vi "sedSpectrometer_flushSamplesEvent_ErrorCode.vi"(8 "error in (no error)":errorcluster) -> (0 "error out":errorcluster, 3 "function return":i32)   [LabVIEW 2016, in "SALLV_sedSpectrometer.lvlib"]
doc: "int sedSpectrometer_shm_flushSamplesEvent_ErrorCodeLV();"
uses:
  SALLV_sedSpectrometer.lvlib
  SALLV_sedSpectrometer.so
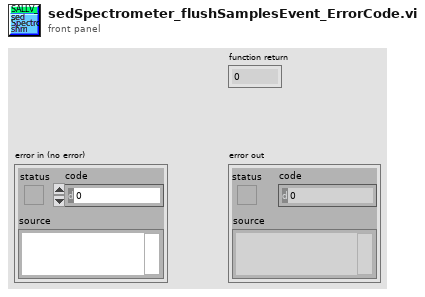
[diagram p1: front panel]
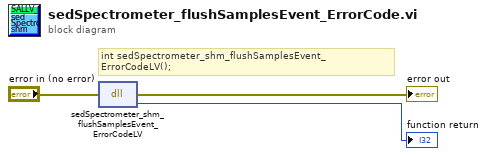
[diagram p0: block diagram]
diagram:
  # "int sedSpectrometer_shm_flushSamplesEvent_ErrorCodeLV();"
  n1 = dll-call lib="home/harini/TCS/ts_sallv_sedSpectrometer/SALLV_sedSpectrometer.*" fn="sedSpectrometer_shm_flushSamplesEvent_ErrorCodeLV"(error in="error in (no error)") -> (error out=→"error out":errorcluster, →"function return":i32)  [unwired: 2 in, 1 out]
